vi "Select Channel.vi"(8 "error in (no error)":errorcluster, 10 "Channel":i32, 11 "UI ACTOR in":refnum<class "UI ACTOR.lvclass">) -> (0 "error out":errorcluster, 3 "UI ACTOR out":refnum<class "UI ACTOR.lvclass">)   [LabVIEW 2020, in "UI ACTOR.lvlib" / "UI ACTOR.lvclass"]
uses:
  UI ACTOR.lvclass
  UI ACTOR.lvclass/UI ACTOR.ctl
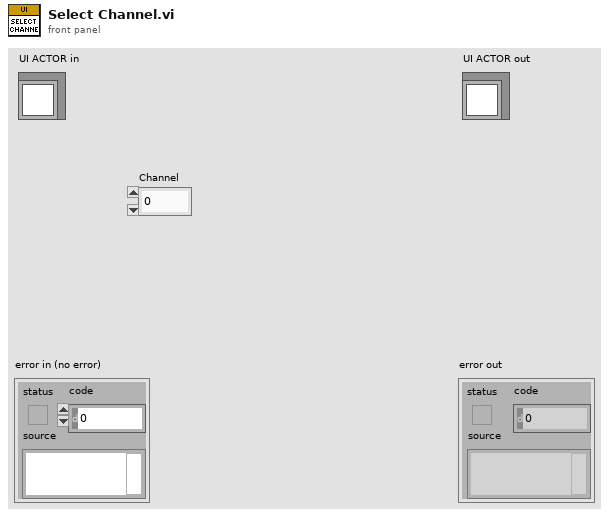
[diagram p1: front panel]
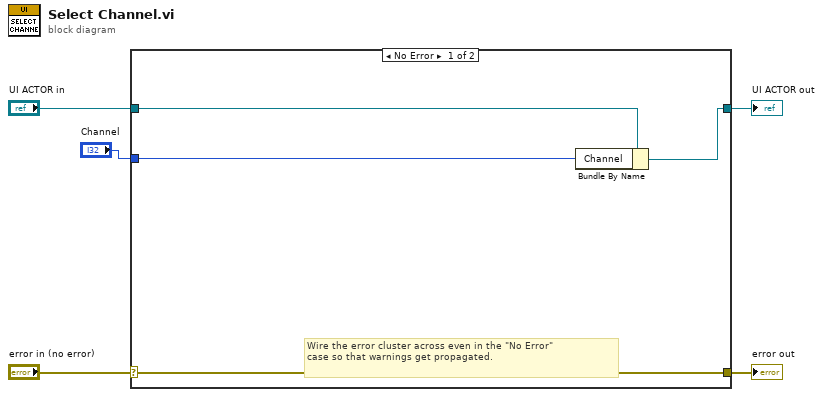
[diagram p0: block diagram]
diagram:
  n1 = case shown="No Error" "error in (no error)" {
    selector: "error in (no error)" -> [w9 w11]
    tunnel: [w9 w11] -> w4
    tunnel: [w6 w10] -> w2
    tunnel: "UI ACTOR in" -> [w8 w10]
    tunnel: "Channel" -> [w7 _]
    frame No Error {
      # "Wire the error cluster across even in the \"No Error\"\ncase so that warnings get propagated."
      n2 = Bundle By Name(cluster=w8, "Channel"=w7) -> (w6:refnum<class "UI ACTOR.lvclass">)
    }
    frame Error {
    }
  }
  "error out" <- w4
  "UI ACTOR out" <- w2
